vi "VISION_LABVIEW.vi"() -> ()   [LabVIEW 2021]
uses:
  <vilib>/userdefined/High Color/IMAQdx.ctl
  <vilib>/MakerHub/LINX/Public/Peripherals/Digital/Digital Write 1 Chan.vi
  <vilib>/MakerHub/LINX/Public/Peripherals/Digital/Digital Write N Chans.vi
  <vilib>/MakerHub/LINX/Private/Local IO/LinxDigitalWrite.vi
  <vilib>/MakerHub/LINX/Public/Utilities/Check Channel.vi
  <vilib>/MakerHub/LINX/Public/Utilities/Open Serial.vi
  <vilib>/MakerHub/LINX/Private/Utilties/Generate Error.vi
  <vilib>/vision/driver/NI_Vision_Acquisition_Software.lvlib
  <resource>/objmgr/imaqdx.rc
  <vilib>/vision/NI_Vision_Development_Module.lvlib
  <vilib>/MakerHub/LINX/LMH-LINX.lvlib
panel:
  in  "Digital Output Channel":u8=13
  out "Loop Rate (Hz)":u32
  in  "stop":bool
  in  "Serial Port":refnum<visa-resource-name>
  in  "Bucar":bool
  out "posision \"y\" del objeto":sgl
  out "posicion \"x \" del objeto":sgl
  in  "Match Feature Mode 2":u32(ring) items=["Color and Shape", "Color", "Shape"]
  in  "Color Score Weight 2":sgl=500.0 min=0 max=1000 format="%.2f"
  in  "Minimum Contrast 2":i32=10
  in  "Search Strategy 2":u32(ring) items=["Conservative", "Balance", "Aggressive", "Very Aggressive"]
  in  "Color Sensitivity 2":u32(ring)=2 items=["Low Sensitivity", "Medium Sensitivity", "High Sensitivity"]
  in  "Match Mode 2":u32(ring) items=["Shift Invariant", "Rotation Invariant"]
  in  "Minimum Score":sgl=700.0
  in  "Nb of Matches":i32=4
  in  "Subpixel Accuracy 2":bool
  in  "Aprende":bool
  in  "X Step Size":i32=1
  in  "Y Step Size":i32=1
  out "Image":T1(plugin-control)
  out "VIDEO1":T1(plugin-control)
  in  "y":bool
  in  "VideoMode":u32
  in  "Camera Name":T2
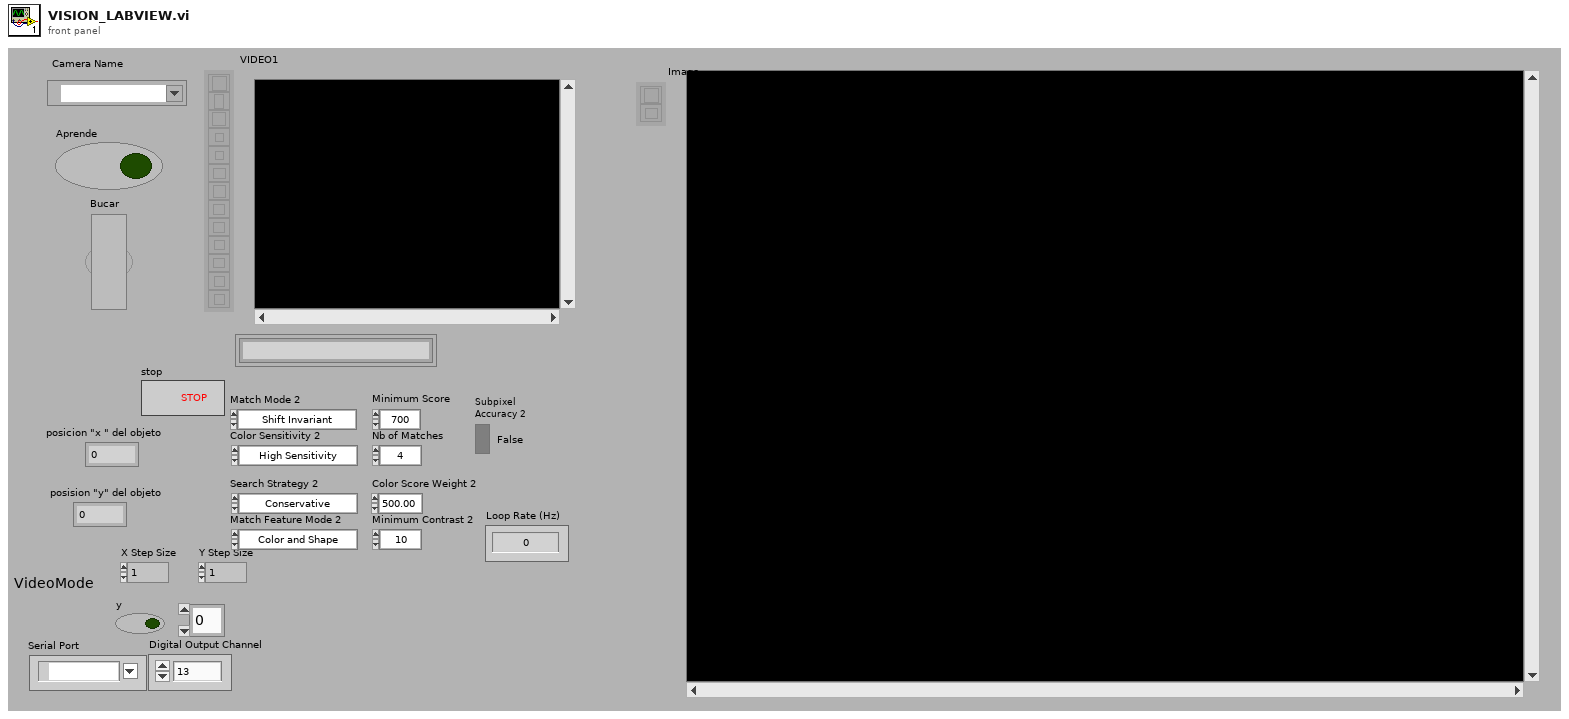
[diagram p1: front panel]
types:
  T1 = typedef "IMAQ Image.ctl" = refnum<image>
  T2 = typedef "IMAQdx.ctl" = refnum<k21>
  T3 = typedef "LMH-LINX.lvlib/LINX Ref.ctl" = cluster{"IO":T4, "Interface":T5, "LINX Device Config":T6}
  T4 = typedef "LMH-LINX.lvlib/Platform.ctl" = enum16{"Remote", "Local"}
  T5 = typedef "LMH-LINX.lvlib/Interface.ctl" = enum16{"Serial", "TCP"}
  T6 = typedef "LMH-LINX.lvlib/Device.lvlib/LINX Device Config.ctl" = cluster{"Interface":T5, "COM Port":refnum<visa-resource-name>, "TCP Configuration":T7, "Device Family":u8, "Device ID":u8, "Device Name":string, "TCP Ref":refnum<k5>, "Channels":T8}
  T7 = typedef "LMH-LINX.lvlib/Device.lvlib/TCP Config.ctl" = cluster{"IP Address":string, "Port":u16}
  T8 = typedef "LMH-LINX.lvlib/Channels.ctl" = cluster{"DI":u8[], "DO":u8[], "AI":u8[], "AO":u8[], "PWM":u8[], "QE":u8[], "UART":u8[], "I2C 2":u8[], "SPI":u8[], "CAN":u8[], "Servo":u8[], "AI Ref (V)":dbl, "AI Resolution (Bits)":u8, "AO Ref (V)":dbl, "AO Resolution (Bits)":u8}
  T9 = cluster{"Position":cluster{"x":sgl, "y":sgl}, "Angle":sgl, "Scale":sgl, "Score":sgl, "Bounding Box":cluster{"x":sgl, "y":sgl}[]}[]
  T10 = cluster{"Position":cluster{"x":sgl, "y":sgl}, "Angle":sgl, "Scale":sgl, "Score":sgl, "Bounding Box":cluster{"x":sgl, "y":sgl}[]}
  T11 = typedef "Image Type" = u32
  T12 = cluster{"Global Rectangle":i32[], "Contours":cluster{"Contour Type":u32, "ROI Type":u32, "Points":i32[]}[]}
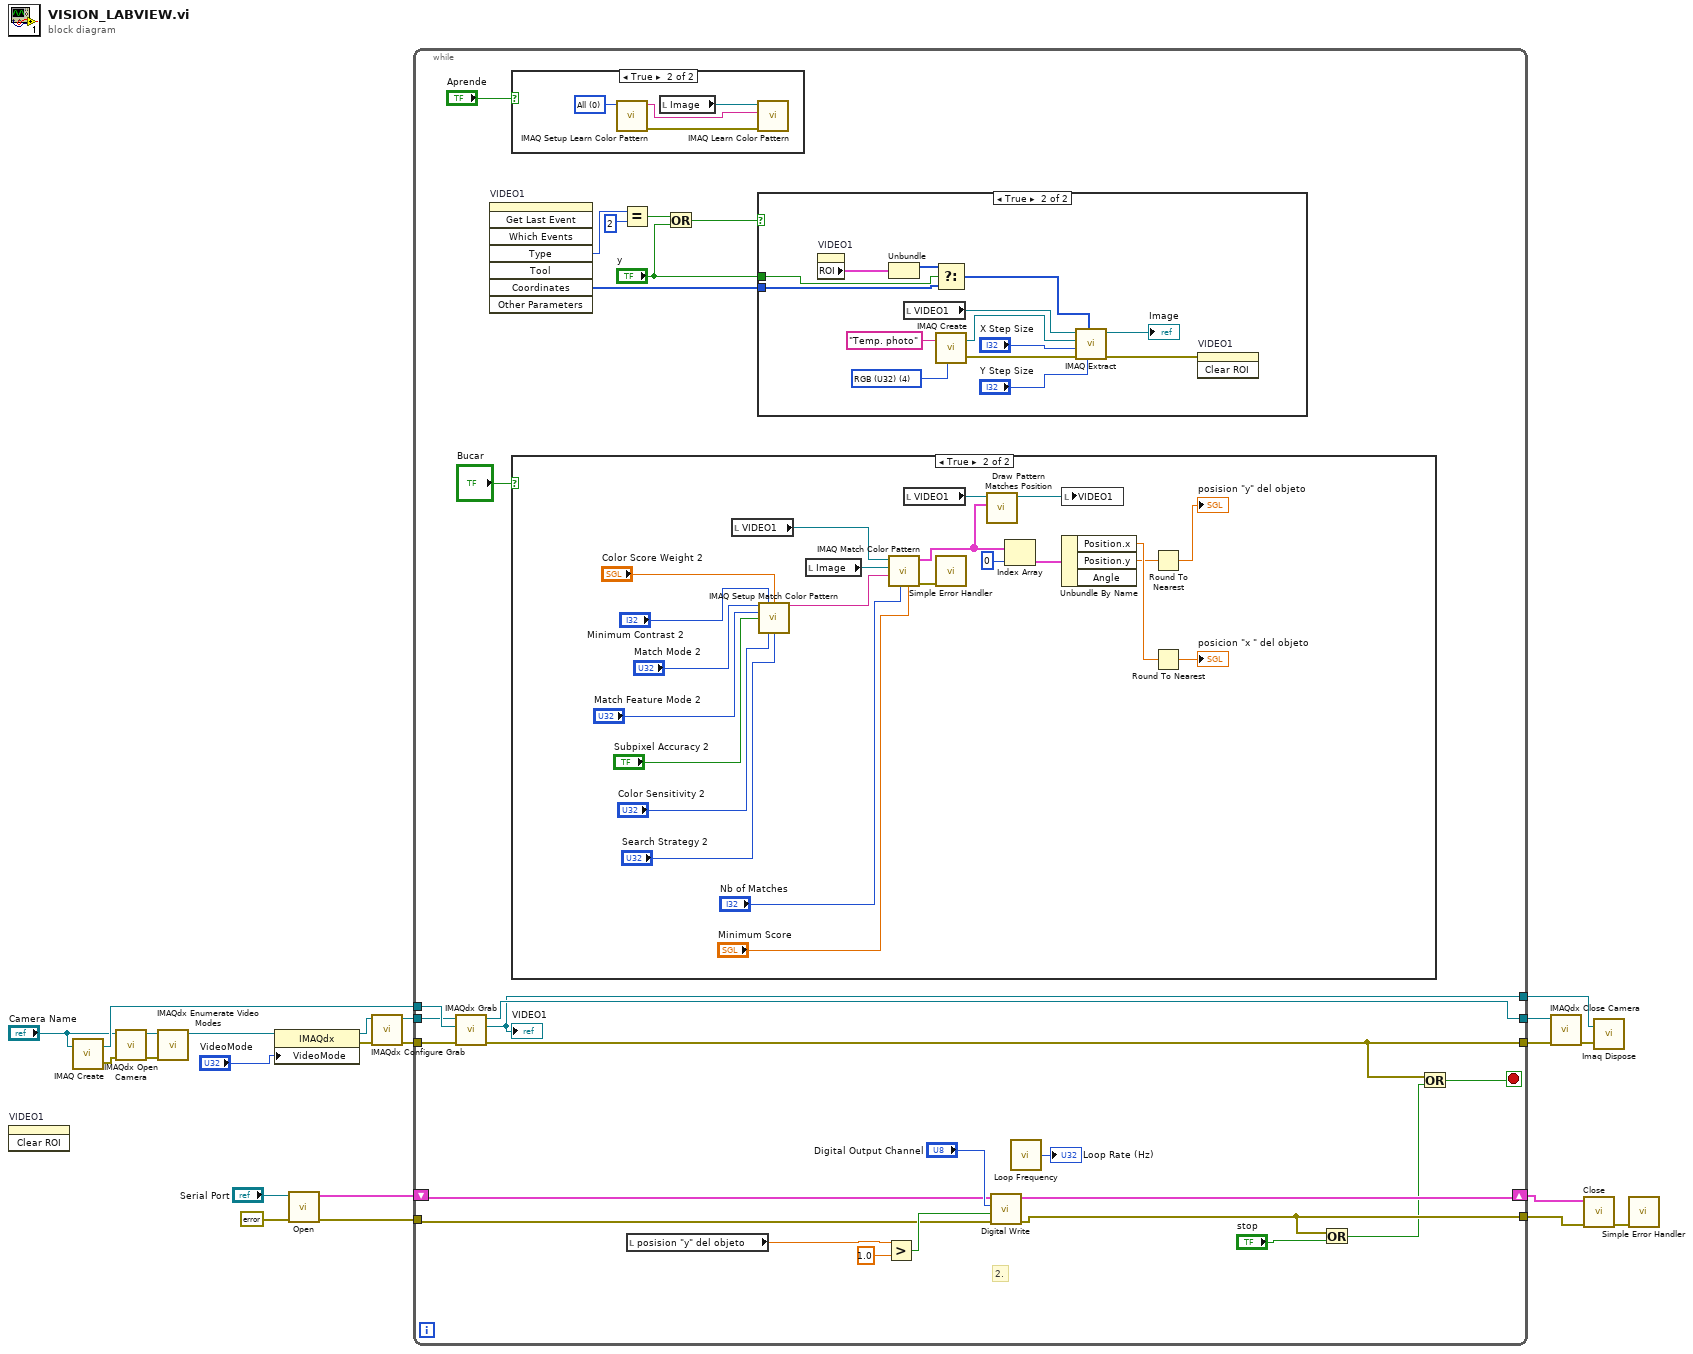
[diagram p0: block diagram]
diagram:
  n1 = invoke on="VIDEO1" class="ImageControl" method="Clear ROI"() -> ()  [unwired: 3 in, 3 out]
  n2 = call "IMAQ Create"("Image Name"="Camera Name") -> ("New Image"=w15:T1, "error out"=w16:errorcluster)  [unwired: 3 in, 1 out]
  n3 = call <vilib>:"IMAQdx Open Camera.vi"("error in"=w16, "Session In"="Camera Name") -> ("error out"=w21:errorcluster, "Session Out"=w22:T2)  [unwired: 1 in, 7 out]
  n4 = call <vilib>:"IMAQdx Enumerate Video Modes.vi"("error in"=w21, "Session In"=w22) -> ("Session Out"=w18:T2)  [unwired: 6 in, 3 out]
  n5 = property class="IMAQdx"(reference=w18, "VideoMode"="VideoMode") -> (reference out=w20:T2, error out=w19:errorcluster)  [unwired: 1 in]
  n6 = call-poly <vilib>:"Open.vi"("Error In"=errorcluster {"status"=FALSE, "code"=0, "source"=""}, "Serial Port"="Serial Port") -> ("Error Out"=w4:errorcluster, "LINX Resource"=w5:T3)  [unwired: 7 in, 1 out]
  n7 = call <vilib>:"IMAQdx Configure Grab.vi"("error in"=w19, "Session In"=w20) -> ("error out"=w13:errorcluster, "Session Out"=w14:T2)  [unwired: 1 in, 7 out]
  n8 = while {
    tunnel: w15 -> [w48]
    tunnel: w14 -> [w47]
    tunnel: w13 -> [w46]
    tunnel: [w40] -> w11
    tunnel: [w45] -> w12
    tunnel: [w26] -> w10
    shift-right: [w29] -> w2
    shift-left: w5 -> [w31]
    tunnel: w4 -> [w30]
    tunnel: [w27] -> w1
    stop <- w25 stop-if-true
    # "2."
    n9 = call <vilib>:"IMAQdx Grab.vi"("error in"=w46, "Image In"=w48, "Session In"=w47) -> ("error out"=w26:errorcluster, "Image Out"=w40:T1, "Session Out"=w45:T2)  [unwired: 1 in, 5 out]
    "VIDEO1" <- w40
    n10 = invoke on="VIDEO1" class="ImageControl" method="Get Last Event"() -> ("Type"=w38:i32, "Coordinates"=w39:i32[])  [unwired: 8 in, 6 out]
    n11 = case shown="True" "Aprende" {
      frame False {
      }
      frame True {
        w51 = u32 0 items=["All", "Shift Information", "Rotation Information"] ("Learn Mode")
        n12 = call "IMAQ Setup Learn Color Pattern"("Learn Mode"=w51) -> ("error out"=w50:errorcluster, "Learn Color Pattern Setup Data"=w49:string)  [unwired: 9 in]
        n13 = local read "Image"() -> (w52:T1)
        n14 = call "IMAQ Learn Color Pattern"("error in (no error)"=w50, "Learn Color Pattern Setup Data"=w49, "Image"=w52) -> ()  [unwired: 7 in, 2 out]
      }
    }
    n15 = case shown="True" "Bucar" {
      frame False {
      }
      frame True {
        n16 = local read "VIDEO1"() -> (w75:T1)
        n17 = call "IMAQ Setup Match Color Pattern"("Match Mode"="Match Mode 2", "Minimum Contrast"="Minimum Contrast 2", "Color Score Weight"="Color Score Weight 2", "Match Feature Mode"="Match Feature Mode 2", "Subpixel Accuracy"="Subpixel Accuracy 2", "Color Sensitivity"="Color Sensitivity 2", "Search Strategy"="Search Strategy 2") -> ("Match Color Pattern Setup Data"=w88:string)  [unwired: 7 in, 1 out]
        n18 = local read "Image"() -> (w74:T1)
        n19 = call "IMAQ Match Color Pattern"("Minimum Match Score"="Minimum Score", "Number of Matches Requested"="Nb of Matches", "Match Color Pattern Setup Data"=w88, "Template Image"=w74, "Image"=w75) -> ("error out"=w87:errorcluster, "Matches"=w71:T9)  [unwired: 4 in, 1 out]
        n20 = local read "VIDEO1"() -> (w85:T1)
        n21 = call <vilib>:"Simple Error Handler.vi"("error in (no error)"=w87) -> ()  [unwired: 4 in, 5 out]
        n22 = call "Draw Pattern Matches Position.vi"("Matches"=w71, "Image"=w85) -> ("Image Out"=w86:T1)  [unwired: 9 out]
        n23 = Index Array(array=w71, index=0) -> (element=w72:T10)
        n24 = local write "VIDEO1"(w86) -> ()
        n25 = Unbundle By Name(w72) -> ("Position.x"=w70:sgl, "Position.y"=w68:sgl)  [unwired: 1 out]
        n26 = Round To Nearest(number=w68) -> (nearest integer value=→"posision \"y\" del objeto":sgl)
        n27 = Round To Nearest(number=w70) -> (nearest integer value=→"posicion \"x \" del objeto":sgl)
      }
    }
    n28 = Equal?(x=w38, y=2) -> (x = y?=w43:bool)
    n29 = local read "posision \"y\" del objeto"() -> (w23:sgl)
    n30 = Or(x=w43, y="y") -> (x .or. y?=w42:bool)
    n31 = case shown="True" w42 {
      tunnel: "y" -> [_ w66]
      tunnel: w39 -> [_ w58]
      frame False {
      }
      frame True {
        w61 = T11 4 items=["Grayscale (U8)", "Grayscale (I16)", "Grayscale (SGL)", "Complex (CSG)", "RGB (U32)", "HSL (U32)", "RGB (U64)", "Grayscale (U16)"] ("Image Type")
        n32 = property on="VIDEO1" class="ImageControl"() -> ("ROI"=w59:T12)  [unwired: 2 in, 2 out]
        n33 = Unbundle(w59) -> ("Global Rectangle"=w60:i32[])  [unwired: 1 out]
        n34 = local read "VIDEO1"() -> (w57:T1)
        n35 = Select(t=w60, s=w66, f=w58) -> (s? t:f=w65:i32[])
        n36 = call "IMAQ Create"("Image Name"="Temp. photo", "Image Type"=w61) -> ("New Image"=w64:T1, "error out"=w63:errorcluster)  [unwired: 3 in]
        n37 = call "IMAQ Extract"("Y Step Size"="Y Step Size", "Optional Rectangle"=w65, "error in (no error)"=w63, "X Step Size"="X Step Size", "Image Dst"=w64, "Image Src"=w57) -> ("error out"=w56:errorcluster, "Image Dst Out"=→"Image":T1)  [unwired: 4 in]
        n38 = invoke on="VIDEO1" class="ImageControl" method="Clear ROI"(error in=w56) -> ()  [unwired: 2 in, 3 out]
      }
    }
    n39 = Greater?(x=w23, y=1.0) -> (0:w33:bool)
    n40 = call-poly <vilib>:"Digital Write.vi"("Error In"=w30, "Output Value"=w33, "DO Channel"="Digital Output Channel", "LINX Resource"=w31) -> ("Error Out"=w27:errorcluster, "LINX Resource"=w29:T3)  [unwired: 6 in]
    n41 = call <vilib>:"Loop Frequency.vi"() -> ("Loop Rate (Hz)"=→"Loop Rate (Hz)":u32)
    n42 = Or(x=w27, y="stop") -> (x .or. y?=w24:bool)
    n43 = Or(x=w26, y=w24) -> (x .or. y?=w25:bool)
  }
  n44 = call <vilib>:"IMAQdx Close Camera.vi"("error in"=w10, "Session In"=w12) -> ("error out"=w9:errorcluster)  [unwired: 9 out]
  n45 = call <vilib>:"Close.vi"("Error In"=w1, "LINX Resource"=w2) -> ("Error Out"=w3:errorcluster)  [unwired: 9 in]
  n46 = call "Imaq Dispose"("Image"=w11, "error in (no error)"=w9) -> ()  [unwired: 4 in, 1 out]
  n47 = call <vilib>:"Simple Error Handler.vi"("error in (no error)"=w3) -> ()  [unwired: 4 in, 5 out]
